vi "Data_Concentric Circles.vi"(10 "# of circles":i32=2, 11 "# of points":i32=1000) -> (1 "Classes":i32[](array[numeric]), 3 "Data":dbl[][](array[numeric]))   [LabVIEW 2009]
uses:
  <vilib>/Analysis/NI_AALBase.lvlib
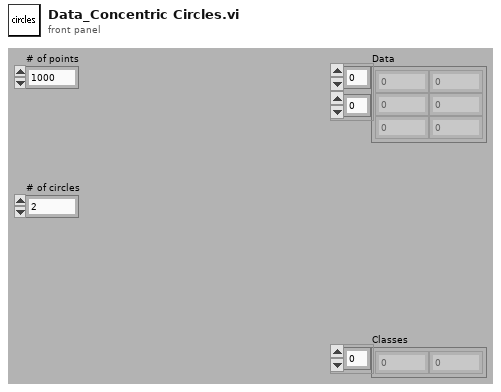
[diagram p1: front panel]
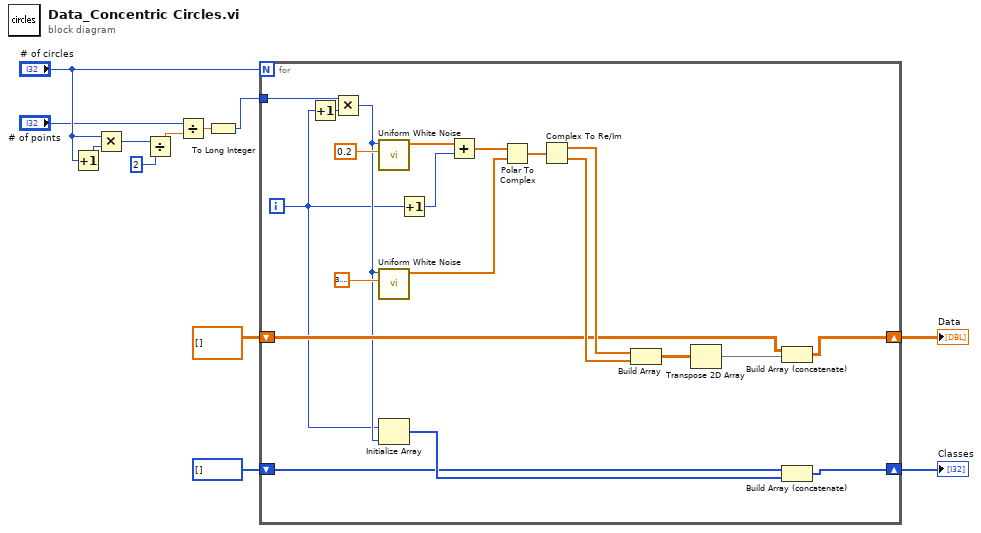
[diagram p0: block diagram]
diagram:
  n1 = Increment(x="# of circles") -> (x+1=w6:i32)
  n2 = Multiply(x="# of circles", y=w6) -> (x*y=w3:i32)
  n3 = Divide(x=w3, y=2) -> (x/y=w2:dbl)
  n4 = Divide(x="# of points", y=w2) -> (x/y=w8:dbl)
  n5 = To Long Integer(number=w8) -> (32bit integer=w7:i32)
  n6 = for {
    N: "# of circles" -> [_]
    shift-right: [w20] -> w11
    shift-left: dbl[][] [] -> [w21]
    shift-right: [w17] -> w10
    shift-left: i32[] [] -> [w18]
    tunnel: w7 -> [w13]
    i -> [w15]
    n7 = Increment(x=w15) -> (x+1=w14:i32)
    n8 = Multiply(x=w13, y=w14) -> (x*y=w16:i32)
    n9 = call <vilib>:"Uniform White Noise.vi"("amplitude"=0.2, "samples"=w16) -> ("uniform white noise"=w30:dbl[])  [unwired: 8 in, 1 out]
    n10 = call <vilib>:"Uniform White Noise.vi"("amplitude"=3.141592653589793, "samples"=w16) -> ("uniform white noise"=w27:dbl[])  [unwired: 8 in, 1 out]
    n11 = Initialize Array(w15, w16) -> (w19:i32[])
    n12 = Increment(x=w15) -> (x+1=w29:i32)
    n13 = Add(x=w30, y=w29) -> (x+y=w28:dbl[])
    n14 = Polar To Complex(1:w27, 2:w28) -> (0:w26:cdb[])
    n15 = Complex To Re/Im(x + iy=w26) -> (x=w25:dbl[], y=w24:dbl[])
    n16 = Build Array(w25, w24) -> (w23:dbl[][])
    n17 = Transpose 2D Array(2D array=w23) -> (transposed array=w22:dbl[][])
    n18 = Build Array (concatenate)(w21, w22) -> (w20:dbl[][])
    n19 = Build Array (concatenate)(w18, w19) -> (w17:i32[])
  }
  "Classes" <- w10
  "Data" <- w11
